vi "Initialize Custom Device Settings.vi"(8 "error in":errorcluster, 10 "Compiled Settings":variant, 11 "Custom Device Settings in":T2={"instrument handle"="Dev1", "NIDMM"={"Name"="", "Properties"={"ResourceName"="", "Model"="", "ScanPeriod(ms)"=0.0, "ResolutionDigits"=0.0, "ACMaxFrequency"=0.0, "ACMinFrequency"=0.0, "TargetOS"="", "TargetRate"=0.0}, "Channels"={"Mode[]"=[], "ActiveMode[]"=[], "DeviceStatus[]"=[], "Heartbeat[]"=[]}, "Sections"={"Voltage[]"=[], "Current[]"=[]}}}) -> (0 "error out":errorcluster, 1 "ChannelRefs":T1, 3 "Custom Device Settings out":T2={"instrument handle"="Dev1", "NIDMM"={"Name"="", "Properties"={"ResourceName"="", "Model"="", "ScanPeriod(ms)"=0.0, "ResolutionDigits"=0.0, "ACMaxFrequency"=0.0, "ACMinFrequency"=0.0, "TargetOS"="", "TargetRate"=0.0}, "Channels"={"Mode[]"=[], "ActiveMode[]"=[], "DeviceStatus[]"=[], "Heartbeat[]"=[]}, "Sections"={"Voltage[]"=[], "Current[]"=[]}}})   [LabVIEW 2026, in "NIDMM Engine.lvlib" / "NIDMM Engine.lvclass"]
uses:
  NIDMM Engine.lvclass
  NIDMM Engine.lvclass/NIDMM Engine.ctl
  Shared/CustomDeviceSettings.ctl
  Shared/GroupedChannelRefs.ctl
  Shared/GroupedChannel.ctl
  Shared/GroupSettings.ctl
  Shared/ChannelGroups.ctl
  Shared/Compiled.Settings.ctl
  Types/TargetSettings.ctl
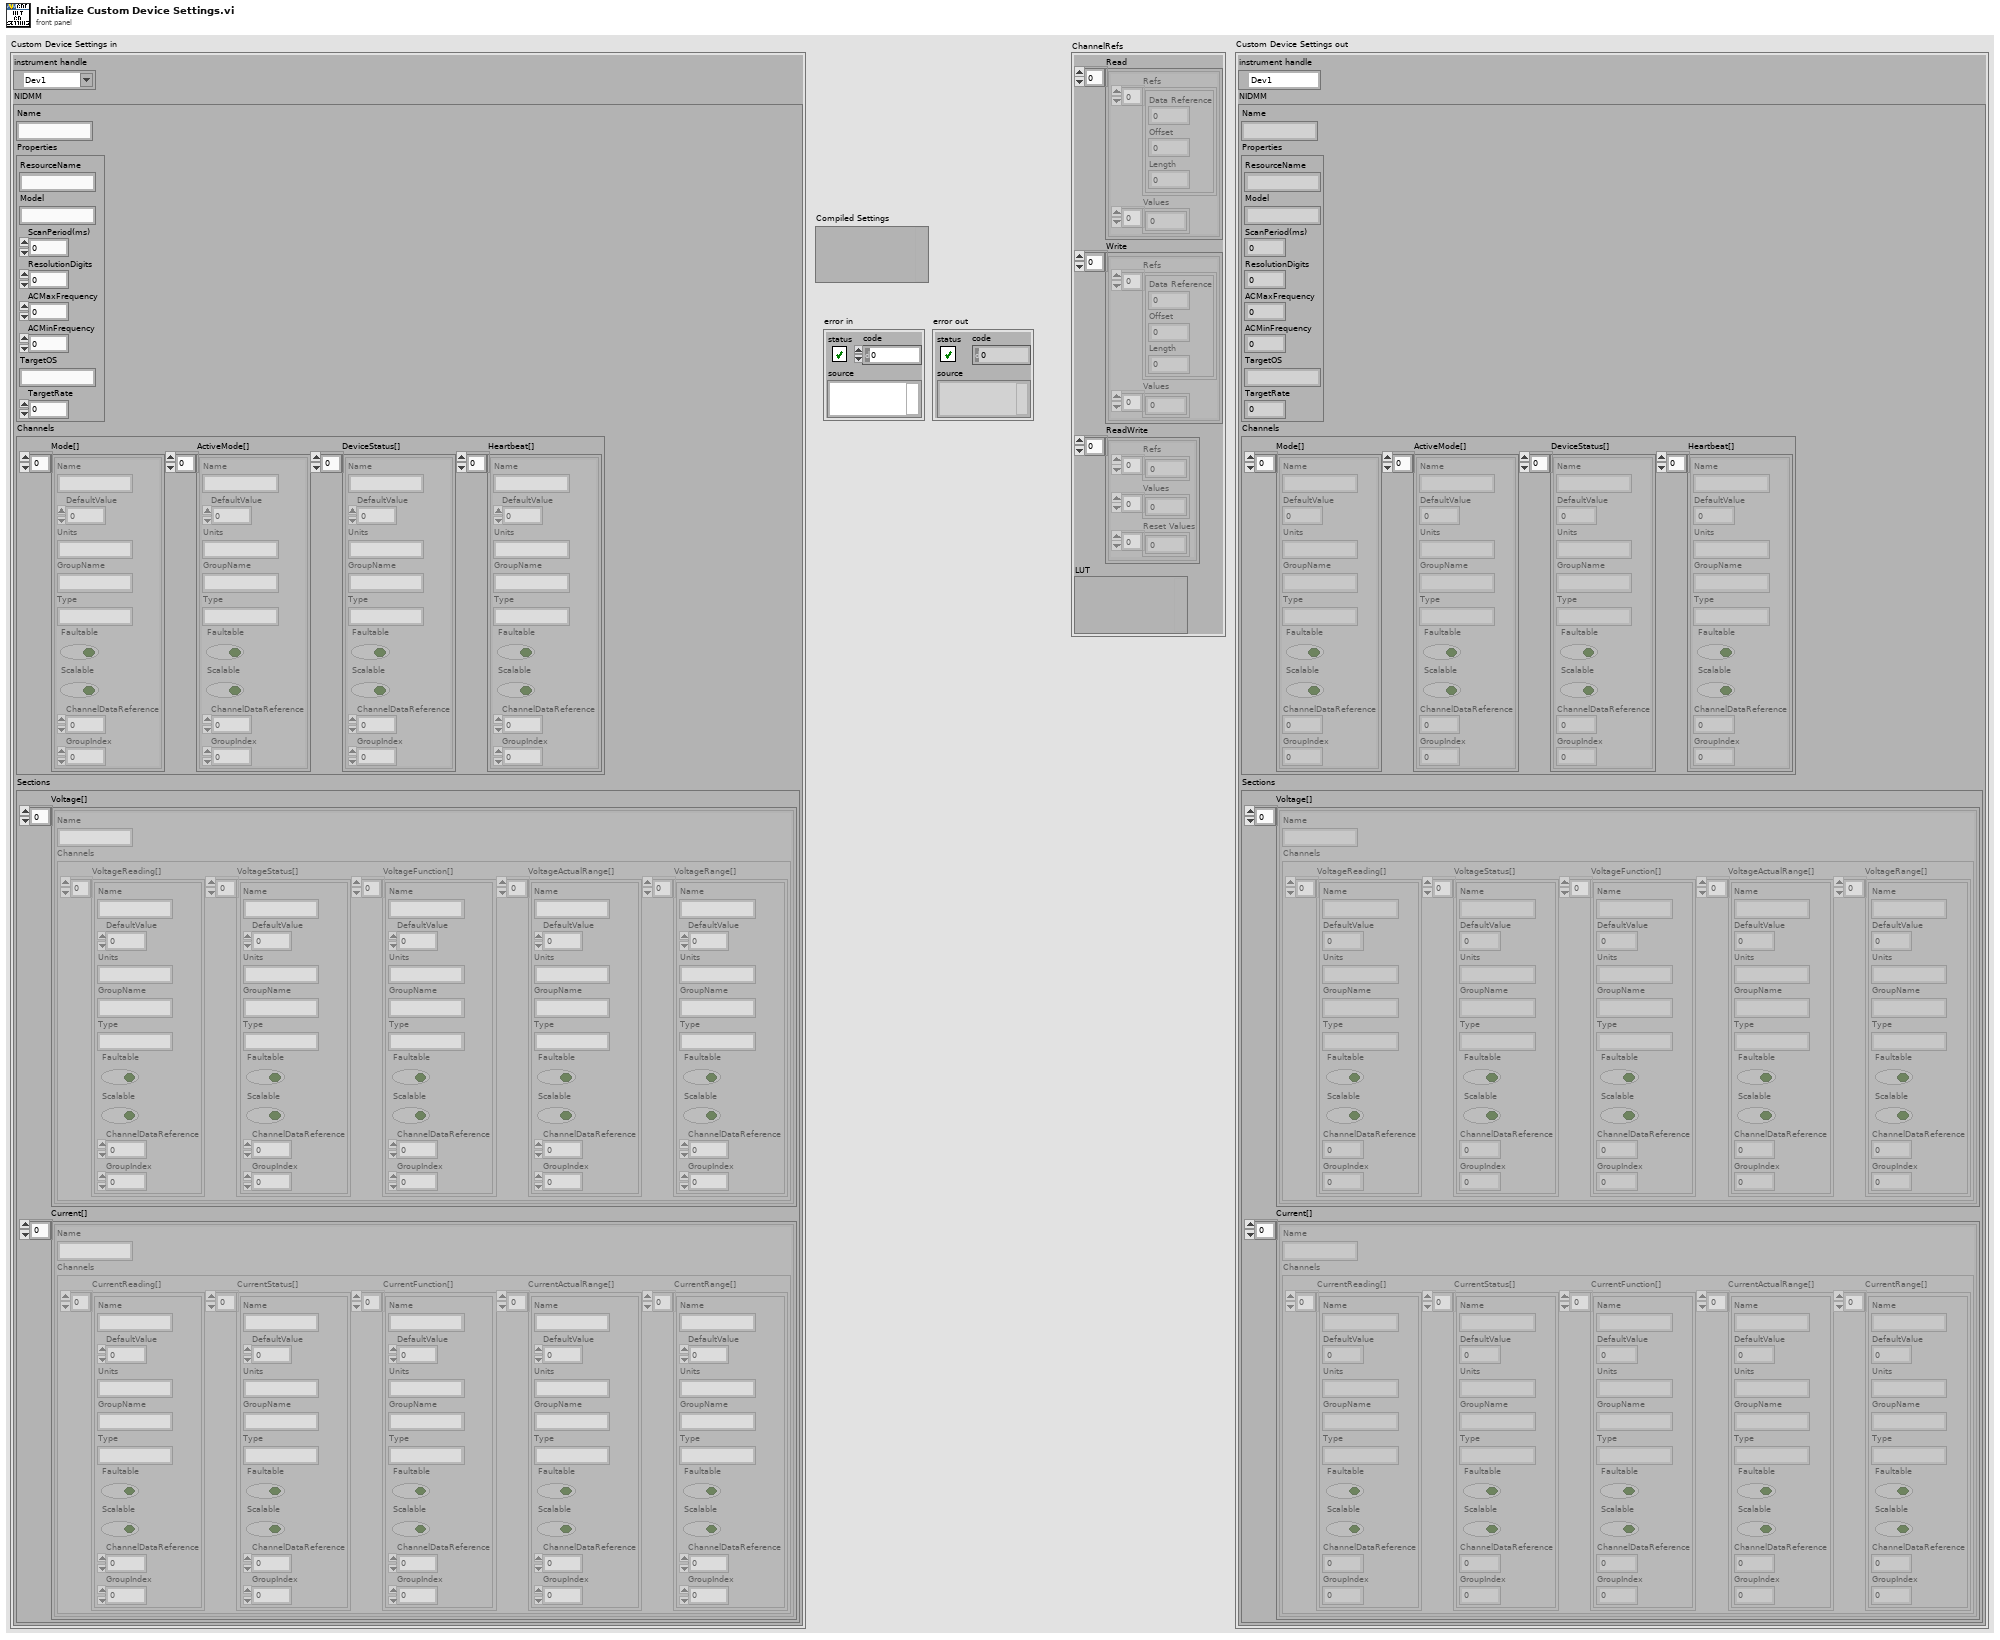
[diagram p1: front panel]
types:
  T1 = typedef "GroupedChannelRefs.ctl" = cluster{"Read":cluster{"Refs":cluster{"Data Reference":i32, "Offset":u64, "Length":u64}[], "Values":dbl[]}[], "Write":cluster{"Refs":cluster{"Data Reference":i32, "Offset":u64, "Length":u64}[], "Values":dbl[]}[], "ReadWrite":cluster{"Refs":i32[], "Values":dbl[], "Reset Values":dbl[]}[], "LUT":variant}
  T2 = typedef "NIDMM Engine.lvlib/NIDMM Engine.lvclass/TargetSettings.ctl" = cluster{"instrument handle":refnum<k15>, "NIDMM":T3}
  T3 = typedef "CustomDeviceSettings.ctl" = cluster{"Name":string, "Properties":cluster{"ResourceName":string, "Model":string, "ScanPeriod(ms)":dbl, "ResolutionDigits":dbl, "ACMaxFrequency":dbl, "ACMinFrequency":dbl, "TargetOS":string, "TargetRate":dbl}, "Channels":cluster{"Mode[]":cluster{"Name":string, "DefaultValue":dbl, "Units":string, "GroupName":string, "Type":string, "Faultable":bool, "Scalable":bool, "ChannelDataReference":i32, "GroupIndex":i32}[], "ActiveMode[]":cluster{"Name":string, "DefaultValue":dbl, "Units":string, "GroupName":string, "Type":string, "Faultable":bool, "Scalable":bool, "ChannelDataReference":i32, "GroupIndex":i32}[], "DeviceStatus[]":cluster{"Name":string, "DefaultValue":dbl, "Units":string, "GroupName":string, "Type":string, "Faultable":bool, "Scalable":bool, "ChannelDataReference":i32, "GroupIndex":i32}[], "Heartbeat[]":cluster{"Name":string, "DefaultValue":dbl, "Units":string, "GroupName":string, "Type":string, "Faultable":bool, "Scalable":bool, "ChannelDataReference":i32, "GroupIndex":i32}[]}, "Sections":cluster{"Voltage[]":cluster{"Name":string, "Channels":cluster{"VoltageReading[]":cluster{"Name":string, "DefaultValue":dbl, "Units":string, "GroupName":string, "Type":string, "Faultable":bool, "Scalable":bool, "ChannelDataReference":i32, "GroupIndex":i32}[], "VoltageStatus[]":cluster{"Name":string, "DefaultValue":dbl, "Units":string, "GroupName":string, "Type":string, "Faultable":bool, "Scalable":bool, "ChannelDataReference":i32, "GroupIndex":i32}[], "VoltageFunction[]":cluster{"Name":string, "DefaultValue":dbl, "Units":string, "GroupName":string, "Type":string, "Faultable":bool, "Scalable":bool, "ChannelDataReference":i32, "GroupIndex":i32}[], "VoltageActualRange[]":cluster{"Name":string, "DefaultValue":dbl, "Units":string, "GroupName":string, "Type":string, "Faultable":bool, "Scalable":bool, "ChannelDataReference":i32, "GroupIndex":i32}[], "VoltageRange[]":cluster{"Name":string, "DefaultValue":dbl, "Units":string, "GroupName":string, "Type":string, "Faultable":bool, "Scalable":bool, "ChannelDataReference":i32, "GroupIndex":i32}[]}}[], "Current[]":cluster{"Name":string, "Channels":cluster{"CurrentReading[]":cluster{"Name":string, "DefaultValue":dbl, "Units":string, "GroupName":string, "Type":string, "Faultable":bool, "Scalable":bool, "ChannelDataReference":i32, "GroupIndex":i32}[], "CurrentStatus[]":cluster{"Name":string, "DefaultValue":dbl, "Units":string, "GroupName":string, "Type":string, "Faultable":bool, "Scalable":bool, "ChannelDataReference":i32, "GroupIndex":i32}[], "CurrentFunction[]":cluster{"Name":string, "DefaultValue":dbl, "Units":string, "GroupName":string, "Type":string, "Faultable":bool, "Scalable":bool, "ChannelDataReference":i32, "GroupIndex":i32}[], "CurrentActualRange[]":cluster{"Name":string, "DefaultValue":dbl, "Units":string, "GroupName":string, "Type":string, "Faultable":bool, "Scalable":bool, "ChannelDataReference":i32, "GroupIndex":i32}[], "CurrentRange[]":cluster{"Name":string, "DefaultValue":dbl, "Units":string, "GroupName":string, "Type":string, "Faultable":bool, "Scalable":bool, "ChannelDataReference":i32, "GroupIndex":i32}[]}}[]}}
  T4 = typedef "Compiled.Settings.ctl" = cluster{"NIDMM":T3, "Channel Groups":T5}
  T5 = typedef "ChannelGroups.ctl" = cluster{"Channel Refs":T1, "Group Settings":T6[]}
  T6 = typedef "GroupSettings.ctl" = cluster{"Name":string, "Type":enum16{"Output/Write", "Input/Read", "Input/ReadWrite"}, "Channel Settings":T7[]}
  T7 = typedef "GroupedChannel.ctl" = cluster{"Name":string, "TypeName":string, "ChannelProperties":variant}
  T8 = enum16{"Output/Write", "Input/Read", "Input/ReadWrite"}
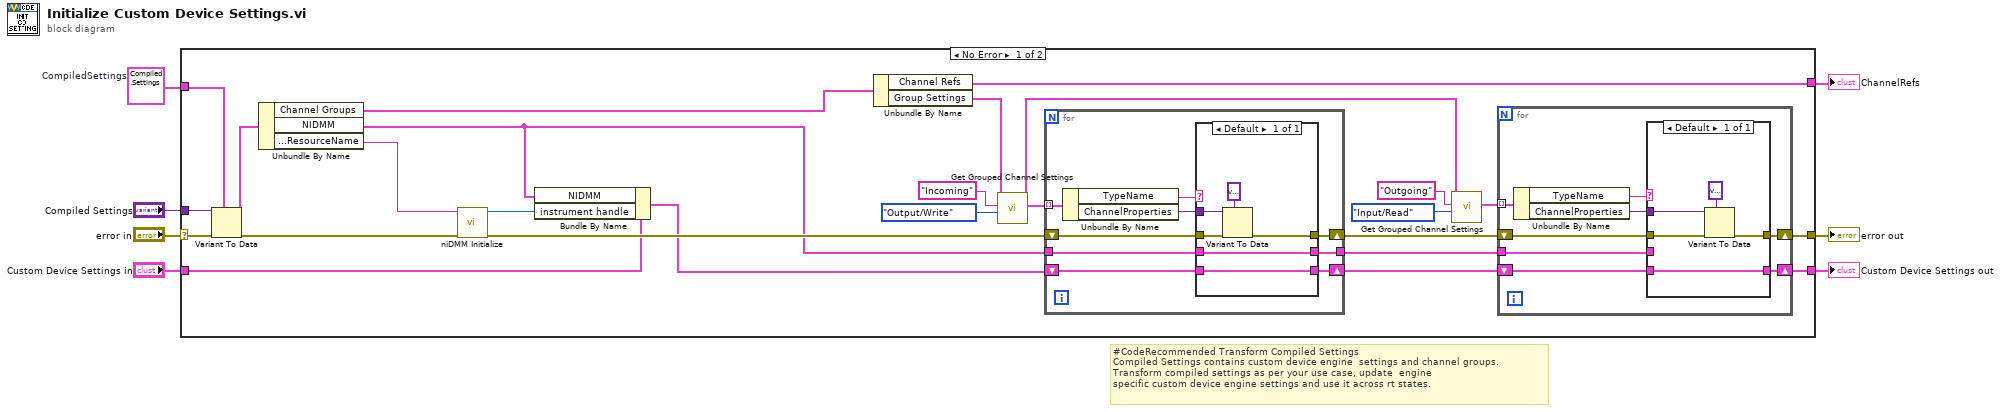
[diagram p0: block diagram]
diagram:
  w1 = T4 {"NIDMM"={"Name"="", "Properties"={"ResourceName"="", "Model"="", "ScanPeriod(ms)"=0.0, "ResolutionDigits"=0.0, "ACMaxFrequency"=0.0, "ACMinFrequency"=0.0, "TargetOS"="", "TargetRate"=0.0}, "Channels"={"Mode[]"=[], "ActiveMode[]"=[], "DeviceStatus[]"=[], "Heartbeat[]"=[]}, "Sections"={"Voltage[]"=[], "Current[]"=[]}}, "Channel Groups"={"Channel Refs"={"Read"=[], "Write"=[], "ReadWrite"=[], "LUT"=variant}, "Group Settings"=[]}}  # CompiledSettings
  # "#CodeRecommended Transform Compiled Settings\nCompiled Settings contains custom device engine  settings and channel groups.\nTransform compiled settings as per your use case, update  engine\nspecific custom device engine settings and use it across rt states."
  n1 = case shown="No Error" "error in" {
    selector: "error in" -> [w32 w63]
    tunnel: [w33 w63] -> w6
    tunnel: [w29 w62] -> w5
    tunnel: "Custom Device Settings in" -> [w12 w62]
    tunnel: "Compiled Settings" -> [w31 _]
    tunnel: [w30 _] -> w2
    tunnel: w1 -> [w28 _]
    frame No Error {
      n2 = Variant To Data(error in=w32, type=w28, Variant=w31) -> (data=w13:T4, error out=w15:errorcluster)
      n3 = Unbundle By Name(w13) -> ("Channel Groups"=w8:T5, "NIDMM"=w10:T3, "NIDMM.Properties.ResourceName"=w16:string)
      n4 = call <instrlib>:"niDMM Initialize.vi"("error in (no error)"=w15, "Instrument Descriptor"=w16) -> ("error out"=w14:errorcluster, "instrument handle out"=w9:refnum<k15>)  [unwired: 8 in]
      n5 = Bundle By Name(cluster=w12, "NIDMM"=w10, "instrument handle"=w9) -> (w11:T2)
      n6 = Unbundle By Name(w8) -> ("Channel Refs"=w30:T1, "Group Settings"=w26:T6[])
      n7 = call "Get Grouped Channel Settings.vi"("Type"=T8."Output/Write", "Group Name"="Incoming", "Group Settings"=w26) -> ("Channel Settings"=w23:T7[], "Name based Group Settings"=w20:T6[])  [unwired: 6 in, 1 out]
      n8 = for {
        tunnel: w23 -> [w40] mode=indexing
        tunnel: w10 -> [w37]
        shift-right: [w36] -> w17
        shift-left: w11 -> [w35]
        tunnel: [w34] -> w18
        shift-right: [w41] -> w27
        shift-left: w14 -> [w42]
        n9 = Unbundle By Name(w40) -> ("TypeName"=w39:string, "ChannelProperties"=w38:variant)
        n10 = case "Incoming" shown="Default" w39 {
          tunnel: w38 -> [w44]
          tunnel: w37 -> [w45]
          tunnel: [w46] -> w36
          tunnel: w35 -> [w46]
          tunnel: [w45] -> w34
          tunnel: w42 -> [w48]
          tunnel: [w47] -> w41
          frame Default {
            n11 = Variant To Data(error in=w48, type=variant, Variant=w44) -> (error out=w47:errorcluster)  [unwired: 1 out]
          }
        }
      }
      n12 = call "Get Grouped Channel Settings.vi"("Type"=T8."Input/Read", "Group Name"="Outgoing", "Group Settings"=w20) -> ("Channel Settings"=w19:T7[])  [unwired: 6 in, 2 out]
      n13 = for {
        tunnel: w19 -> [w54] mode=indexing
        tunnel: w18 -> [w51]
        shift-right: [w50] -> w29
        shift-left: w17 -> [w49]
        shift-right: [w55] -> w33
        shift-left: w27 -> [w56]
        n14 = Unbundle By Name(w54) -> ("TypeName"=w53:string, "ChannelProperties"=w52:variant)
        n15 = case "Outgoing" shown="Default" w53 {
          tunnel: w52 -> [w58]
          tunnel: w51 -> [_]
          tunnel: [w59] -> w50
          tunnel: w49 -> [w59]
          tunnel: w56 -> [w61]
          tunnel: [w60] -> w55
          frame Default {
            n16 = Variant To Data(error in=w61, type=variant, Variant=w58) -> (error out=w60:errorcluster)  [unwired: 1 out]
          }
        }
      }
    }
    frame Error {
    }
  }
  "error out" <- w6
  "Custom Device Settings out" <- w5
  "ChannelRefs" <- w2
